vi "CalcArmCurlSpeed.vi"(9 "Curl Speed":dbl, 10 "Elbow Motor":bool, 11 "Shoulder Motor":bool) -> (2 "Elbow Speed":dbl, 3 "Shoulder Speed":dbl)   [LabVIEW 2018]
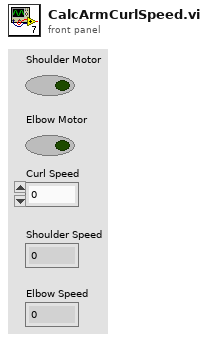
[diagram p1: front panel]
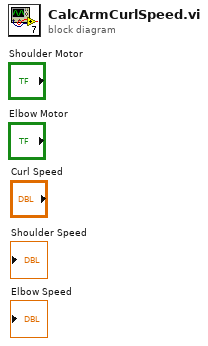
[diagram p0: block diagram]
diagram:
